vi "find_sub_contour.vi"(5 "Pad ROI arrays":i32[][][](array[numeric]), 7 "Y Resolution":i32, 9 "extrinsic":cluster{"extrinsic":dbl[][], "resolution":i32[]}, 10 "Segment Information":T1(array[cluster]), 11 "rectangle corner":dbl[][](array[numeric])) -> (0 "other Y":dbl[](array[numeric]), 1 "other X":dbl[](array[numeric]), 2 "Pad Y":dbl[](array[numeric]), 3 "Pad X":dbl[](array[numeric]))   [LabVIEW 2017]
panel:
  out "Pad ROI arrays 2":i32[][][](array[numeric])
  out "Array":dbl[](array[numeric])
  out "max corner":dbl[][](array[numeric])
  in  "max index":dbl
  in  "max area":dbl
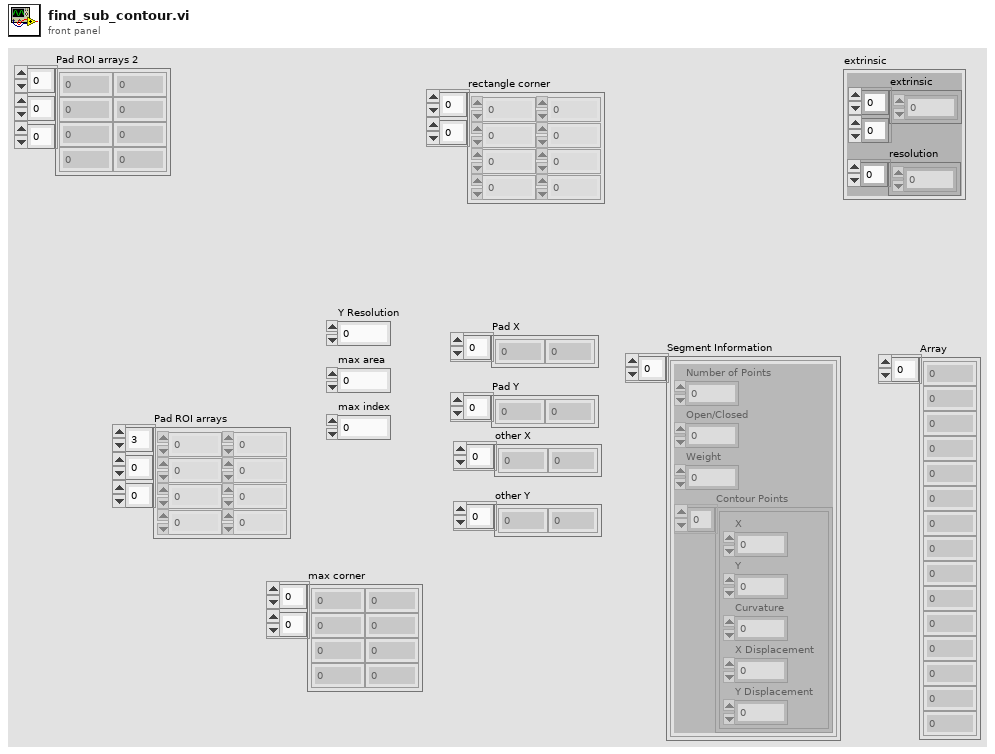
[diagram p1: front panel]
types:
  T1 = cluster{"Number of Points":i32, "Open/Closed":i32, "Weight":dbl, "Contour Points":cluster{"X":dbl, "Y":dbl, "Curvature":dbl, "X Displacement":dbl, "Y Displacement":dbl}[]}[]
  T2 = cluster{"X":dbl, "Y":dbl, "Curvature":dbl, "X Displacement":dbl, "Y Displacement":dbl}[]
  T3 = cluster{"Number of Points":i32, "Open/Closed":i32, "Weight":dbl, "Contour Points":cluster{"X":dbl, "Y":dbl, "Curvature":dbl, "X Displacement":dbl, "Y Displacement":dbl}[]}
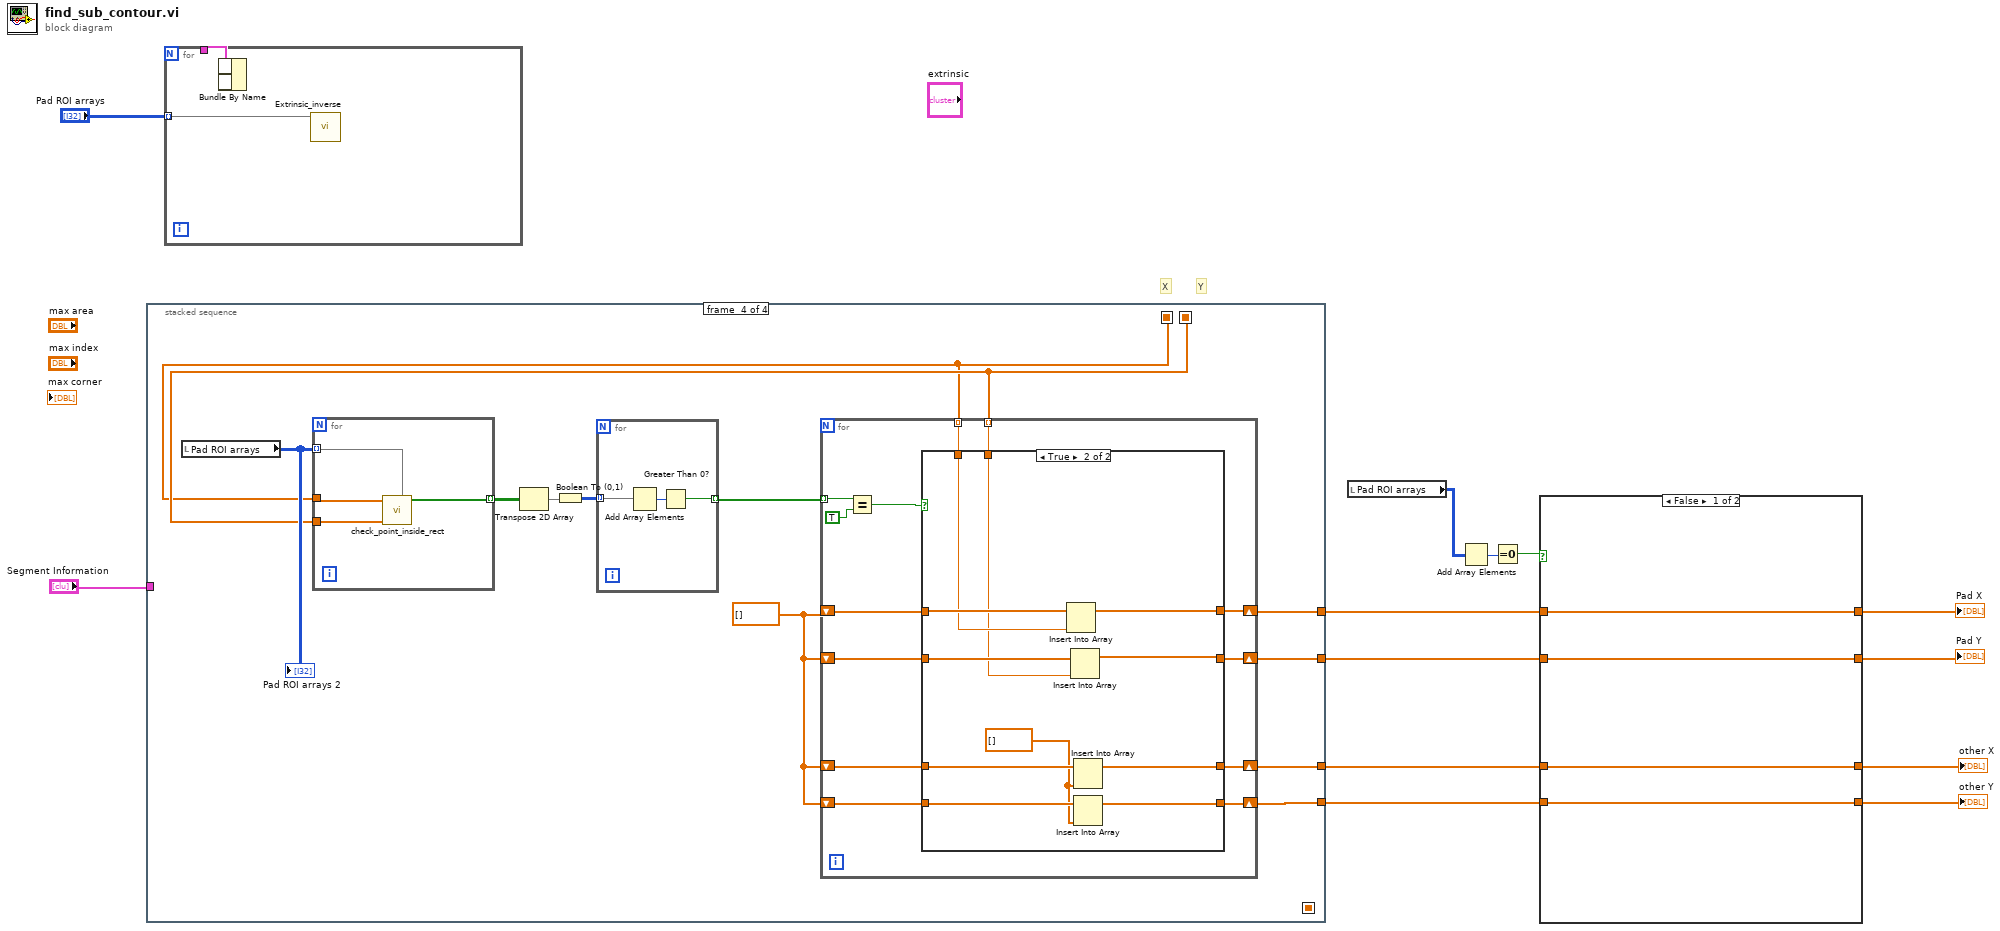
[diagram p0: block diagram]
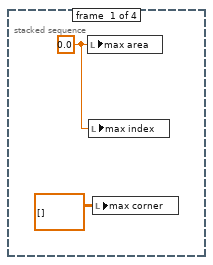
[diagram p3: hidden frame]
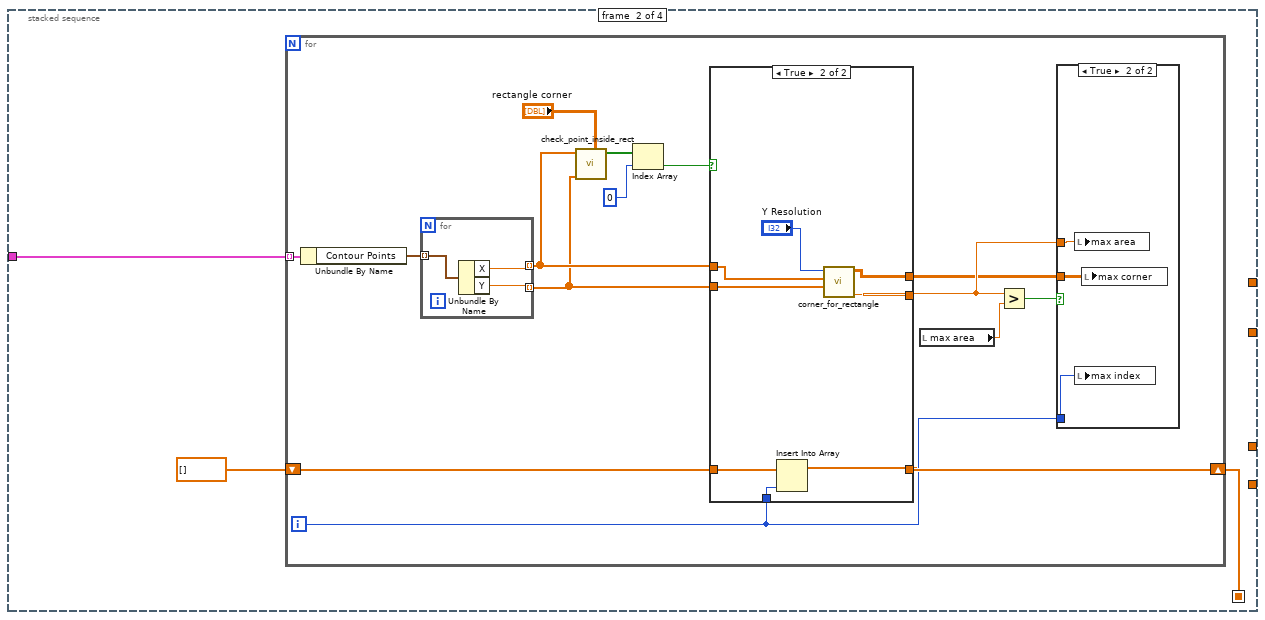
[diagram p4: hidden frame]
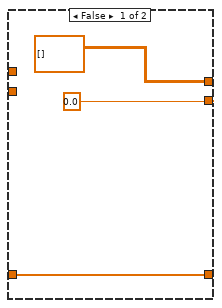
[diagram p6: hidden frame]
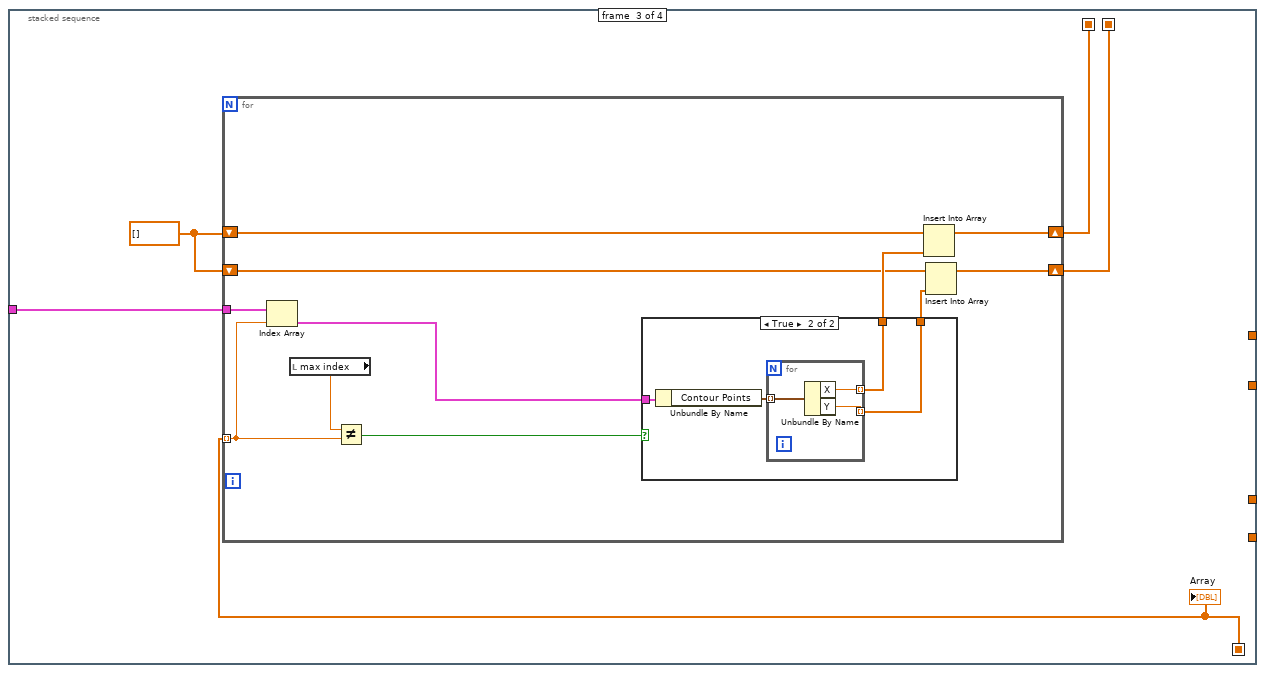
[diagram p7: hidden frame]
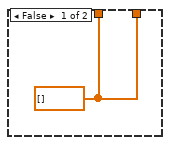
[diagram p8: hidden frame]
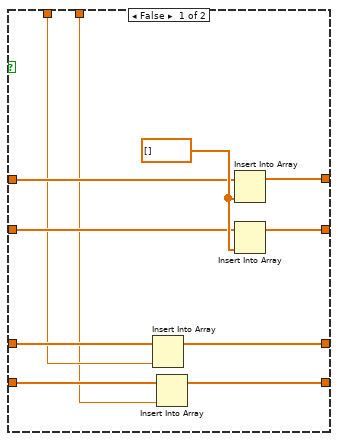
[diagram p9: hidden frame]
diagram:
  # "Y"
  # "X"
  n1 = stacked-sequence {
    seq-local: [_ w17 _ _] -> [_ _ w55 _]
    seq-local: [_ _ w53 _] -> [_ _ _ w81]
    seq-local: [_ _ w52 _] -> [_ _ _ w82]
    tunnel: "Segment Information" -> [_ w19 w56 _]
    tunnel: [_ _ _ w79] -> w7
    tunnel: [_ _ _ w78] -> w8
    tunnel: [_ _ _ w77] -> w9
    tunnel: [_ _ _ w76] -> w10
    frame #0 {
      w16 = 0.0
      n2 = local write "max area"(w16) -> ()
      n3 = local write "max index"(w16) -> ()
      n4 = local write "max corner"(dbl[][] [] ("max corner")) -> ()
    }
    frame #1 {
      n5 = for {
        tunnel: w19 -> [w34] mode=indexing
        shift-right: [w25] -> w17
        shift-left: dbl[] [] -> [w26]
        i -> [w24]
        n6 = Unbundle By Name(w34) -> ("Contour Points"=w33:T2)
        n7 = for {
          tunnel: w33 -> [w51] mode=indexing
          tunnel: [w50] -> w28 mode=indexing
          tunnel: [w49] -> w20 mode=indexing
          n8 = Unbundle By Name(w51) -> ("X"=w50:dbl, "Y"=w49:dbl)
        }
        n9 = call "check_point_inside_rect.vi"("rectangle corner"="rectangle corner", "Y"=w20, "X"=w28) -> ("result"=w23:bool[])  [unwired: 8 in]
        n10 = Index Array(array=w23, index=0) -> (element=w22:bool)
        n11 = case shown="True" w22 {
          tunnel: w28 -> [_ w48]
          tunnel: [0.0 w47] -> w30
          tunnel: [dbl[][] [] ("max corner") w46] -> w29
          tunnel: w26 -> [w38 w45]
          tunnel: [w38 w44] -> w25
          tunnel: w24 -> [_ w42]
          tunnel: w20 -> [_ w41]
          frame False {
          }
          frame True {
            n12 = Insert Into Array "Insert Into Array"(array=w45, new element=w42) -> (w44:dbl[])  [unwired: 1 in]
            n13 = call "corner_for_rectangle.vi"("Y"=w41, "X"=w48, "Y Resolution"="Y Resolution") -> ("area"=w47:dbl, "corner"=w46:dbl[][])  [unwired: 6 in, 1 out]
          }
        }
        n14 = local read "max area"() -> (w32:dbl)
        n15 = Greater?(x=w30, y=w32) -> (0:w31:bool)
        n16 = case shown="True" w31 {
          tunnel: w30 -> [_ w37]
          tunnel: w24 -> [_ w36]
          tunnel: w29 -> [_ w35]
          frame False {
          }
          frame True {
            n17 = local write "max area"(w37) -> ()
            n18 = local write "max index"(w36) -> ()
            n19 = local write "max corner"(w35) -> ()
          }
        }
      }
    }
    frame #2 {
      w54 = dbl[] []
      n20 = for {
        tunnel: w56 -> [w60]
        shift-right: [w65] -> w53
        shift-left: w54 -> [w67]
        shift-right: [w62] -> w52
        shift-left: w54 -> [w64]
        tunnel: w55 -> [w57] mode=indexing
        n21 = Index Array(array=w60, index=w57) -> (element=w59:T3)
        n22 = local read "max index"() -> (w61:dbl)
        n23 = Not Equal?(x=w61, y=w57) -> (x != y?=w58:bool)
        n24 = case shown="True" w58 {
          tunnel: w59 -> [_ w71]
          tunnel: [w68 w70] -> w66
          tunnel: [w68 w69] -> w63
          frame False {
            w68 = dbl[] []
          }
          frame True {
            n25 = Unbundle By Name(w71) -> ("Contour Points"=w72:T2)
            n26 = for {
              tunnel: w72 -> [w75] mode=indexing
              tunnel: [w74] -> w70 mode=indexing
              tunnel: [w73] -> w69 mode=indexing
              n27 = Unbundle By Name(w75) -> ("X"=w74:dbl, "Y"=w73:dbl)
            }
          }
        }
        n28 = Insert Into Array "Insert Into Array"(array=w67, new element=w66) -> (w65:dbl[])  [unwired: 1 in]
        n29 = Insert Into Array(array=w64, new element=w63) -> (w62:dbl[])  [unwired: 1 in]
      }
      "Array" <- w55
    }
    frame #3 {
      w80 = dbl[] []
      n30 = local read "Pad ROI arrays"() -> (w87:i32[][][])
      "Pad ROI arrays 2" <- w87
      n31 = for {
        tunnel: w87 -> [w127] mode=indexing
        tunnel: w82 -> [w129]
        tunnel: w81 -> [w128]
        tunnel: [w126] -> w86 mode=indexing
        n32 = call "check_point_inside_rect.vi"("rectangle corner"=w127, "Y"=w129, "X"=w128) -> ("result"=w126:bool[])  [unwired: 8 in]
      }
      n33 = Transpose 2D Array(2D array=w86) -> (transposed array=w85:bool[][])
      n34 = Boolean To (0,1)(Boolean=w85) -> (0, 1=w84:i16[][])
      n35 = for {
        tunnel: w84 -> [w125] mode=indexing
        tunnel: [w123] -> w83 mode=indexing
        n36 = Add Array Elements(numeric array=w125) -> (sum=w124:i16)
        n37 = Greater Than 0?(x=w124) -> (x > 0?=w123:bool)
      }
      n38 = for {
        tunnel: w83 -> [w100] mode=indexing
        tunnel: w82 -> [w96] mode=indexing
        tunnel: w81 -> [w97] mode=indexing
        shift-right: [w90] -> w76
        shift-left: w80 -> [w91]
        shift-right: [w88] -> w77
        shift-left: w80 -> [w89]
        shift-right: [w94] -> w78
        shift-left: w80 -> [w95]
        shift-right: [w92] -> w79
        shift-left: w80 -> [w93]
        n39 = Equal?(x=w100, y=TRUE) -> (x = y?=w98:bool)
        n40 = case shown="True" w98 {
          tunnel: w97 -> [w102 w121]
          tunnel: w96 -> [w101 w117]
          tunnel: w95 -> [w106 w116]
          tunnel: [w105 w115] -> w94
          tunnel: w93 -> [w104 w114]
          tunnel: [w103 w113] -> w92
          tunnel: w91 -> [w110 w122]
          tunnel: [w109 w120] -> w90
          tunnel: w89 -> [w108 w119]
          tunnel: [w107 w118] -> w88
          frame False {
            w111 = dbl[] []
            n41 = Insert Into Array(array=w106, new element=w102) -> (w105:dbl[])  [unwired: 1 in]
            n42 = Insert Into Array(array=w104, new element=w101) -> (w103:dbl[])  [unwired: 1 in]
            n43 = Insert Into Array "Insert Into Array"(array=w110, new element=w111) -> (w109:dbl[])  [unwired: 1 in]
            n44 = Insert Into Array(array=w108, new element=w111) -> (w107:dbl[])  [unwired: 1 in]
          }
          frame True {
            w112 = dbl[] []
            n45 = Insert Into Array "Insert Into Array"(array=w122, new element=w121) -> (w120:dbl[])  [unwired: 1 in]
            n46 = Insert Into Array(array=w119, new element=w117) -> (w118:dbl[])  [unwired: 1 in]
            n47 = Insert Into Array(array=w116, new element=w112) -> (w115:dbl[])  [unwired: 1 in]
            n48 = Insert Into Array(array=w114, new element=w112) -> (w113:dbl[])  [unwired: 1 in]
          }
        }
      }
    }
  }
  n49 = for {
    tunnel: "Pad ROI arrays" -> [w131] mode=indexing
    tunnel: [w130] -> w1
    n50 = Bundle By Name(w130) -> ()  [unwired: 2 in, 1 out]
    n51 = call "Extrinsic_inverse.vi"("X'"=w131) -> ()  [unwired: 10 in, 1 out]
  }
  n52 = local read "Pad ROI arrays"() -> (w12:i32[][][])
  n53 = Add Array Elements(numeric array=w12) -> (sum=w13:i32)
  n54 = Equal To 0?(x=w13) -> (x = 0?=w11:bool)
  n55 = case shown="False" w11 {
    tunnel: w10 -> [w135 w139]
    tunnel: w9 -> [w134 w138]
    tunnel: w8 -> [w133 w136]
    tunnel: w7 -> [w132 w137]
    tunnel: [w135 w136] -> w6
    tunnel: [w134 w137] -> w5
    tunnel: [w133 w139] -> w4
    tunnel: [w132 w138] -> w3
    frame False {
    }
    frame True {
    }
  }
  "Pad X" <- w6
  "Pad Y" <- w5
  "other X" <- w4
  "other Y" <- w3
